vi "SRTS_Burst_Save2.vi"(7 "XLS ref.":refnum<vi>, 8 "error in":errorcluster, 10 "Burst_Result":T1, 11 "XLS in":refnum<class "XLS.lvclass">=refnum) -> (0 "error out":errorcluster, 2 "Progress":i32, 3 "XLS out":refnum<class "XLS.lvclass">)   [LabVIEW 2017, in "Report_lib.lvlib" / "XLS.lvclass"]
uses:
  XLS.lvclass
  TypeDefs/Burst_Result.ctl
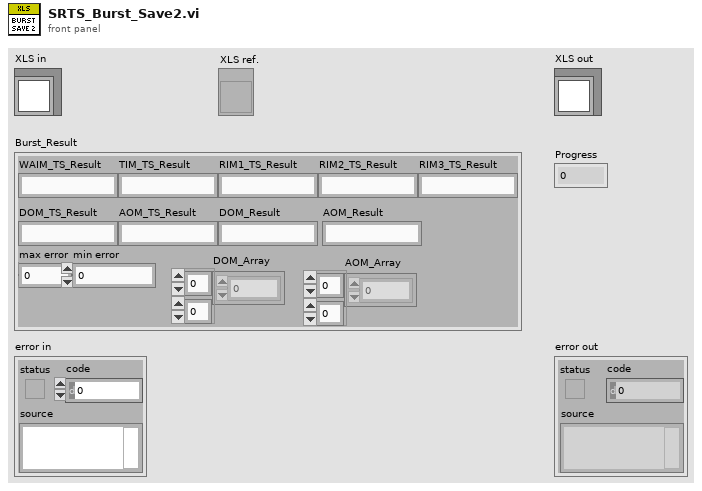
[diagram p1: front panel]
types:
  T1 = typedef "Burst_Result.ctl" = cluster{"WAIM_TS_Result":string, "DOM_TS_Result":string, "AOM_TS_Result":string, "TIM_TS_Result":string, "RIM2_TS_Result":string, "RIM1_TS_Result":string, "RIM3_TS_Result":string, "DOM_Result":string, "AOM_Result":string, "max error":dbl, "min error":dbl, "DOM_Array":dbl[][], "AOM_Array":dbl[][]}
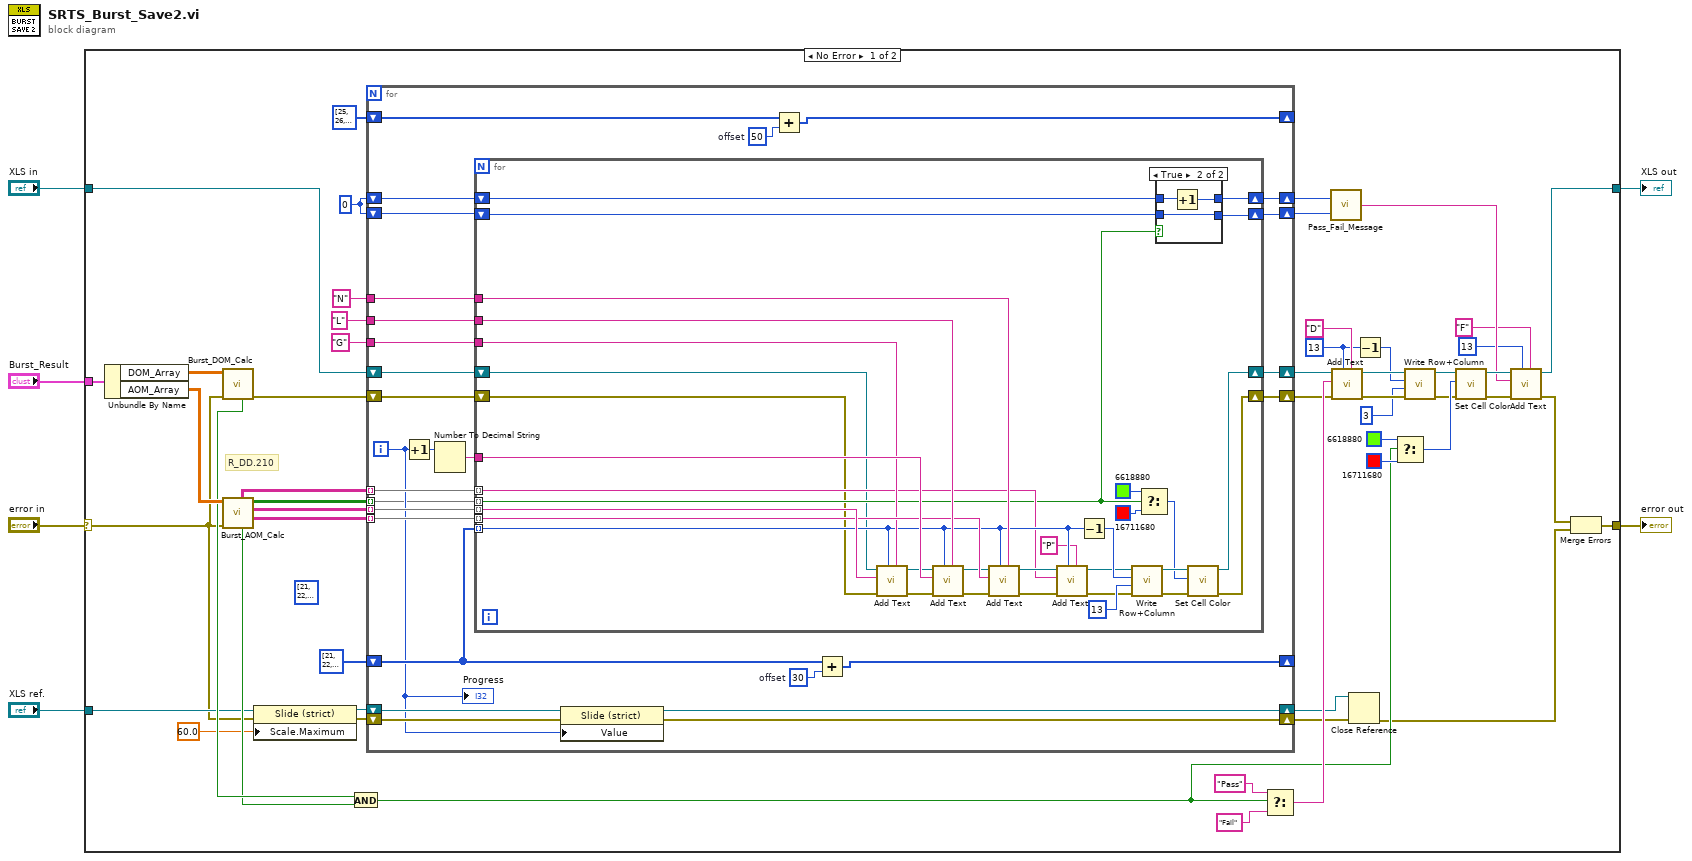
[diagram p0: block diagram]
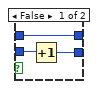
[diagram p2: hidden frame]
diagram:
  n1 = case shown="No Error" "error in" {
    selector: "error in" -> [w21 w127]
    tunnel: [w23 w127] -> w5
    tunnel: [w12 w126] -> w3
    tunnel: "XLS in" -> [w54 w126]
    tunnel: "Burst_Result" -> [w58 _]
    tunnel: "XLS ref." -> [w22 _]
    frame No Error {
      w17 = 0
      w37 = 13 ("Index")
      (unwired) i32[] [21, 22, 23, 24, 29, 30, 31, 32, 37, 38, 39, 40, 45, 46, 47, 48, 53, 54, 55, 56, 61, 62, 63, 64] ("AOM_indexies")
      # "R_DD.210"
      n2 = Unbundle By Name(w58) -> ("DOM_Array"=w57:dbl[][], "AOM_Array"=w56:dbl[][])
      n3 = call "Burst_DOM_Calc.vi"("error in"=w21, "DOM"=w57) -> ("error out"=w55:errorcluster, "DOM_Total"=w29:bool)  [unwired: 5 in, 3 out]
      n4 = call "Burst_AOM_Calc.vi"("error in"=w21, "AOM"=w56) -> ("AOM_Result_Str"=w47:string[][], "AOM_Values"=w48:string[][], "AOM_Result_Bool"=w49:bool[][], "AOM_Total"=w28:bool, "Errors%"=w46:string[][])  [unwired: 4 in, 1 out]
      n5 = property class="Slide (strict)"(reference=w22, error in=w21, "Scale.Maximum"=60.0 ("Scale.Range:Maximum")) -> (reference out=w19:refnum<vi>, error out=w20:errorcluster)
      n6 = And(x=w29, y=w28) -> (x .and. y?=w27:bool)
      n7 = for {
        tunnel: "G" -> [w84]
        shift-right: [w80] -> _
        shift-left: i32[] [25, 26, 27, 28, 33, 34, 35, 36, 41, 42, 43, 44, 49, 50, 51, 52, 57, 58, 59, 60, 65, 66, 67, 68] ("DOM_indexies") -> [w82]
        shift-right: [w77] -> _
        shift-left: i32[] [21, 22, 23, 24, 25, 26, 27, 28, 29, 30, 31, 32, 33, 34, 35, 36, 37, 38, 39, 40, 41, 42, 43, 44] ("AOM_indexies") -> [w79]
        tunnel: w48 -> [w83] mode=indexing
        shift-right: [w76] -> w30
        shift-left: w54 -> [w85]
        shift-right: [w75] -> w31
        shift-left: w55 -> [w86]
        tunnel: "L" -> [w73]
        tunnel: "N" -> [w72]
        tunnel: w47 -> [w71] mode=indexing
        tunnel: w49 -> [w63] mode=indexing
        tunnel: w46 -> [w69] mode=indexing
        shift-right: [w66] -> w25
        shift-left: w19 -> [w68]
        shift-right: [w65] -> w26
        shift-left: w20 -> [w67]
        shift-right: [w60] -> w16
        shift-left: w17 -> [w62]
        shift-right: [w59] -> w15
        shift-left: w17 -> [w61]
        i -> [w64]
        w78 = 30  # offset
        w81 = 50  # offset
        n8 = Increment(x=w64) -> (x+1=w70:i32)
        n9 = Number To Decimal String(number=w70) -> (decimal integer string=w74:string)  [unwired: 1 in]
        n10 = for {
          shift-right: [w102] -> w76
          shift-left: w85 -> [w87]
          shift-right: [w101] -> w75
          shift-left: w86 -> [w88]
          tunnel: w84 -> [w112]
          tunnel: w79 -> [w96] mode=indexing
          tunnel: w83 -> [w117] mode=indexing
          tunnel: w74 -> [w115]
          tunnel: w73 -> [w114]
          tunnel: w72 -> [w107]
          tunnel: w71 -> [w113] mode=indexing
          tunnel: w63 -> [w89] mode=indexing
          tunnel: w69 -> [w94] mode=indexing
          shift-right: [w90] -> w60
          shift-left: w62 -> [w93]
          shift-right: [w91] -> w59
          shift-left: w61 -> [w92]
          n11 = call "Add Text.vi"("Adr"=w112, "Index"=w96, "error in"=w88, "text"=w117, "XLS in"=w87) -> ("error out"=w110:errorcluster, "XLS out"=w111:refnum<class "XLS.lvclass">)  [unwired: 5 in]
          n12 = call "Add Text.vi"("Adr"=w114, "Index"=w96, "error in"=w110, "text"=w115, "XLS in"=w111) -> ("error out"=w108:errorcluster, "XLS out"=w109:refnum<class "XLS.lvclass">)  [unwired: 5 in]
          n13 = call "Add Text.vi"("Adr"=w107, "Index"=w96, "error in"=w108, "text"=w113, "XLS in"=w109) -> ("error out"=w99:errorcluster, "XLS out"=w100:refnum<class "XLS.lvclass">)  [unwired: 5 in]
          n14 = call "Add Text.vi"("Adr"="P", "Index"=w96, "error in"=w99, "text"=w94, "XLS in"=w100) -> ("error out"=w98:errorcluster, "XLS out"=w97:refnum<class "XLS.lvclass">)  [unwired: 5 in]
          n15 = Decrement(x=w96) -> (x-1=w116:i32)
          n16 = call "Write Row+Column.vi"("error in"=w98, "column"=13, "row"=w116, "XLS in"=w97) -> ("error out"=w105:errorcluster, "XLS out"=w106:refnum<class "XLS.lvclass">)  [unwired: 6 in]
          n17 = Select(t=u32 6618880, s=w89, f=u32 16711680) -> (s? t:f=w104:u32)
          n18 = case shown="True" w89 {
            tunnel: w93 -> [w120 w124]
            tunnel: w92 -> [w122 w125]
            tunnel: [w121 w125] -> w91
            tunnel: [w120 w123] -> w90
            frame False {
              n19 = Increment(x=w122) -> (x+1=w121:i32)
            }
            frame True {
              n20 = Increment(x=w124) -> (x+1=w123:i32)
            }
          }
          n21 = call "Set Cell Color.vi"("error in"=w105, "color"=w104, "XLS in"=w106) -> ("error out"=w101:errorcluster, "XLS out"=w102:refnum<class "XLS.lvclass">)  [unwired: 7 in]
        }
        n22 = property class="Slide (strict)"(reference=w68, error in=w67, "Value"=w64) -> (reference out=w66:refnum<vi>, error out=w65:errorcluster)
        n23 = Add(x=w82, y=w81) -> (x+y=w80:i32[])
        n24 = Add(x=w79, y=w78) -> (x+y=w77:i32[])
        "Progress" <- w64
      }
      n25 = Select(t="Pass" ("Adr"), s=w27, f="Fail" ("Adr")) -> (s? t:f=w45:string)
      n26 = call "Pass_Fail_Message.vi"("Failed"=w15, "Passed"=w16) -> ("Result Message"=w10:string)
      n27 = call "Add Text.vi"("Adr"="D", "Index"=w37, "error in"=w31, "text"=w45, "XLS in"=w30) -> ("error out"=w44:errorcluster, "XLS out"=w43:refnum<class "XLS.lvclass">)  [unwired: 5 in]
      n28 = Close Reference(reference=w25, error in (no error)=w26) -> (error out=w24:errorcluster)
      n29 = Decrement(x=w37) -> (x-1=w39:i32)
      n30 = Select(t=u32 6618880, s=w27, f=u32 16711680) -> (s? t:f=w42:u32)
      n31 = call "Write Row+Column.vi"("error in"=w44, "column"=3, "row"=w39, "XLS in"=w43) -> ("error out"=w41:errorcluster, "XLS out"=w40:refnum<class "XLS.lvclass">)  [unwired: 6 in]
      n32 = call "Set Cell Color.vi"("error in"=w41, "color"=w42, "XLS in"=w40) -> ("error out"=w14:errorcluster, "XLS out"=w13:refnum<class "XLS.lvclass">)  [unwired: 7 in]
      n33 = call "Add Text.vi"("Adr"="F", "Index"=13, "error in"=w14, "text"=w10, "XLS in"=w13) -> ("error out"=w11:errorcluster, "XLS out"=w12:refnum<class "XLS.lvclass">)  [unwired: 5 in]
      n34 = Merge Errors(w11, w24) -> (w23:errorcluster)
    }
    frame Error {
    }
  }
  "error out" <- w5
  "XLS out" <- w3
